vi "Open Fault Logs.vi"(8 "error in (no error)":errorcluster, 11 "Fault Monitor in":refnum<class "Fault Monitor.lvclass">) -> (0 "error out":errorcluster, 3 "Fault Monitor out":refnum<class "Fault Monitor.lvclass">)   [LabVIEW 2023, in "Fault Monitor.lvlib" / "Fault Monitor.lvclass"]
uses:
  Library/Fault Monitor.lvclass
  Library/Fault Monitor.lvclass/Fault Monitor.ctl
  builds/Framework/Engine.lvlibp/Engine/Accessors/Read Application Path.vi
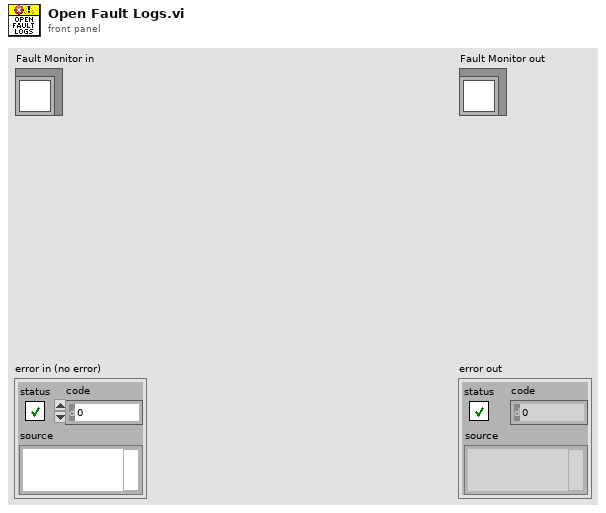
[diagram p1: front panel]
types:
  T1 = enum16{"open", "replace", "create", "open or create", "replace or create", "replace or create with confirmation"}
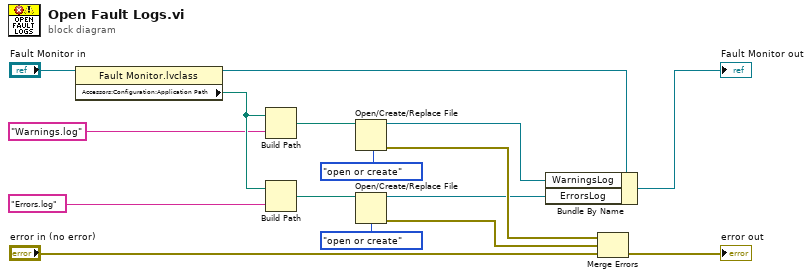
[diagram p0: block diagram]
diagram:
  n1 = property class="Fault Monitor.lvclass"(reference="Fault Monitor in") -> (reference out=w5:refnum<class "Fault Monitor.lvclass">, "Accessors:Configuration:Application Path"=w15:path)  [unwired: 1 in, 1 out]
  n2 = Build Path(base path=w15, name or relative path="Warnings.log") -> (appended path=w11:path)
  n3 = Build Path(base path=w15, name or relative path="Errors.log") -> (appended path=w12:path)
  n4 = Open/Create/Replace File(file path (use dialog)=w11, operation (0:open)=T1."open or create") -> (refnum out=w2:refnum<file>, error out=w6:errorcluster)  [unwired: 4 in, 1 out]
  n5 = Open/Create/Replace File(file path (use dialog)=w12, operation (0:open)=T1."open or create") -> (refnum out=w1:refnum<file>, error out=w7:errorcluster)  [unwired: 4 in, 1 out]
  n6 = Bundle By Name(cluster=w5, "WarningsLog"=w2, "ErrorsLog"=w1) -> (→"Fault Monitor out":refnum<class "Fault Monitor.lvclass">)
  n7 = Merge Errors(w6, w7, "error in (no error)") -> (→"error out":errorcluster)
